vi "))Channel.vi"(0 "channel in":T2, 1 "last element in":bool, 2 "This VI":refnum<vi>, 5 "valid":bool=TRUE, 7 "channelOp":T3, 9 "event priority (norm)":T1=enum."normal priority", 11 "msg in":cluster{"cmd":string, "data":variant}, 12 "abort in":bool, 13 "# event structures":u16=2) -> (3 "last element out":bool, 4 "channel out":T2, 6 "Event Registration Refnum":refnum<event-registration>[](array[refnum]), 8 "This VI out":refnum<vi>, 14 "aborted?":bool)   [LabVIEW 2019, in "Cmd-Data Event Messenger.lvlib"]
uses:
  Cmd-Data Event Messenger.lvlib
  EventMessengerData.lvclass/EventMessengerData.ctl
  Instantiate.vi
  EventMessengerData.lvclass
  <vilib>/event_ctls.llb/usereventprio.ctl
  ))Channel.ctl
  ChannelOp.ctl
  Event Data.ctl
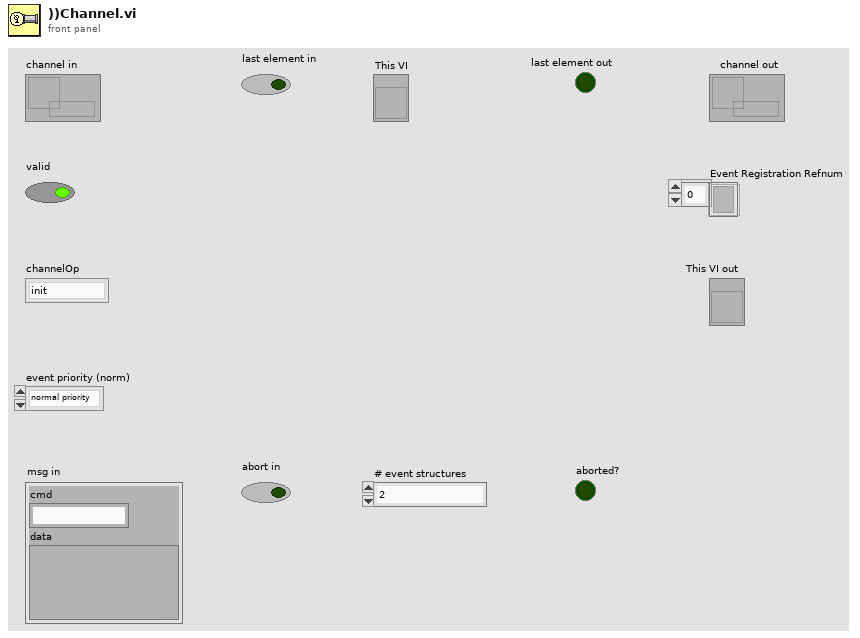
[diagram p1: front panel]
types:
  T1 = typedef "usereventprio.ctl" = enum32{"high priority", "normal priority"}
  T2 = typedef "Cmd-Data Event Messenger.lvlib/))Channel.ctl" = refnum<queue>
  T3 = typedef "Cmd-Data Event Messenger.lvlib/ChannelOp.ctl" = enum16{"init", "write", "register", "replicate", "probe"}
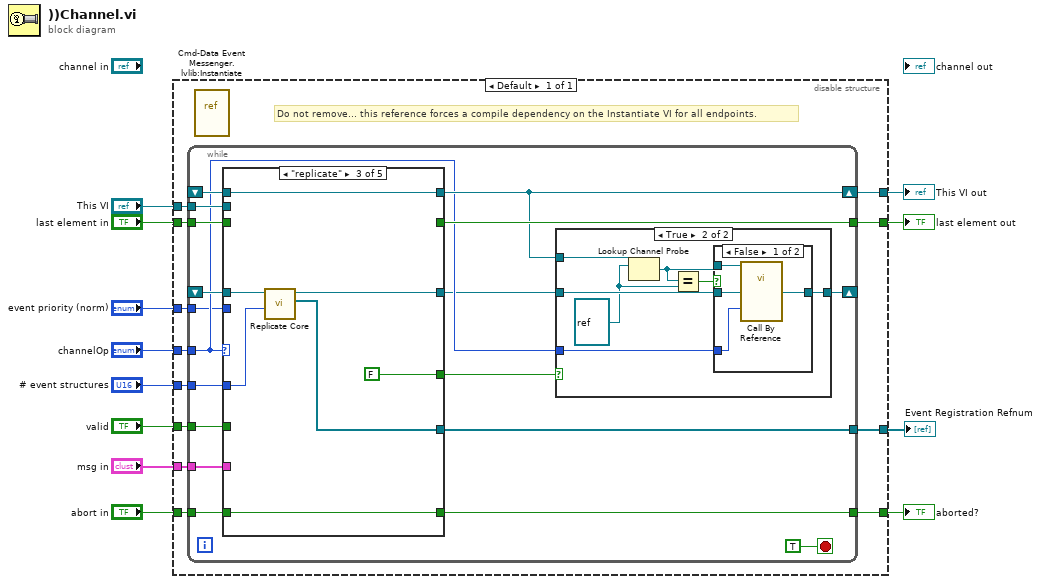
[diagram p0: block diagram]
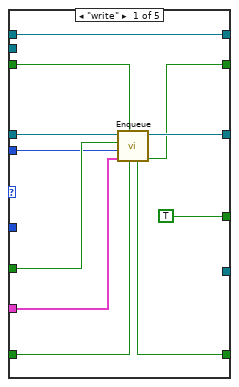
[diagram p4: hidden frame]
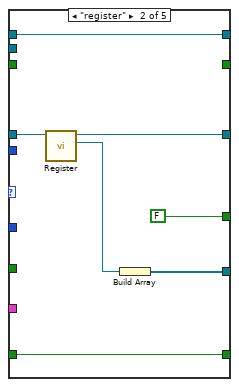
[diagram p5: hidden frame]
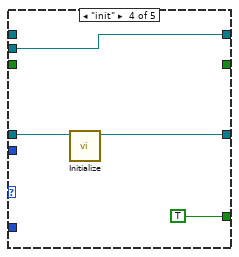
[diagram p6: hidden frame]
diagram:
  n1 = disable-structure shown="Default" {
    disable-tunnel: "msg in" -> [w24]
    disable-tunnel: "channelOp" -> [w23]
    disable-tunnel: "last element in" -> [w22]
    disable-tunnel: [w21] -> w9
    disable-tunnel: "valid" -> [w20]
    disable-tunnel: "abort in" -> [w19]
    disable-tunnel: [w18] -> w6
    disable-tunnel: "This VI" -> [w17]
    disable-tunnel: [w16] -> w4
    disable-tunnel: "event priority (norm)" -> [w15]
    disable-tunnel: "# event structures" -> [w14]
    disable-tunnel: [w13] -> w1
    frame Enabled {
      # "Do not remove... this reference forces a compile dependency on the Instantiate VI for all endpoints."
      n2 = while {
        shift-left: _ -> [w39]
        shift-right: [w32] -> _
        tunnel: w23 -> [w30]
        tunnel: w22 -> [w42]
        tunnel: [w41] -> w21
        tunnel: w20 -> [w38]
        tunnel: w19 -> [w37]
        tunnel: [w36] -> w18
        tunnel: w17 -> [w35]
        shift-right: [w33] -> w16
        shift-left: _ -> [w34]
        tunnel: w24 -> [w29]
        tunnel: [w28] -> w13
        tunnel: w15 -> [w26]
        tunnel: w14 -> [w25]
        stop <- TRUE stop-if-true
        n3 = case shown="\"replicate\"" w30 {
          tunnel: w29 -> [w64 _ _ _ _]
          tunnel: w42 -> [w58 _ _ _ _]
          tunnel: [w57 _ _ _ _] -> w41
          tunnel: [w65 w72 w76 w83 w86] -> w27
          tunnel: w39 -> [w66 w73 w77 w84 w86]
          tunnel: w38 -> [w63 _ _ _ _]
          tunnel: w37 -> [w62 w69 w78 _ _]
          tunnel: [w61 w69 w78 _ _] -> w36
          tunnel: w35 -> [_ _ _ w82 _]
          tunnel: [w60 w71 w80 w82 w85] -> w33
          tunnel: w34 -> [w60 w71 w80 _ w85]
          tunnel: [TRUE ("not an occurrence?") FALSE ("not an occurrence?") FALSE ("not an occurrence?") TRUE _] -> w31
          tunnel: [_ w67 w75 _ _] -> w28
          tunnel: w26 -> [w56 _ _ _ _]
          tunnel: w25 -> [_ _ w74 _ _]
          frame "write" {
            n4 = call "Enqueue.vi"("abort? (F)"=w62, "last element? (F)"=w58, "msg"=w64, "event priority"=w56, "is valid? (T)"=w63, "data in"=w66) -> ("last element?"=w57:bool, "data out"=w65:refnum<class "EventMessengerData.lvclass">, "aborted?"=w61:bool)  [unwired: 3 in]
          }
          frame "register" {
            n5 = call "Register.vi"("data in"=w73) -> ("Event Registration Refnum"=w68:refnum<event-registration>, "data out"=w72:refnum<class "EventMessengerData.lvclass">)  [unwired: 9 in]
            n6 = Build Array(w68) -> (w67:refnum<event-registration>[])
          }
          frame "replicate" {
            n7 = call "Replicate Core.vi"("# event structures"=w74, "data in"=w77) -> ("Event Registration Refnum"=w75:refnum<event-registration>[], "data out"=w76:refnum<class "EventMessengerData.lvclass">)  [unwired: 8 in]
          }
          frame "init" {
            n8 = call "Initialize.vi"("data in"=w84) -> ("data out"=w83:refnum<class "EventMessengerData.lvclass">)  [unwired: 9 in, 1 out]
          }
          frame "probe" {
            # "Probe case only exists to get the This VI Out."
          }
        }
        n9 = case shown="True" w31 {
          tunnel: w33 -> [_ w46]
          tunnel: w27 -> [w43 w49]
          tunnel: [w43 w48] -> w32
          tunnel: w30 -> [_ w47]
          frame False {
          }
          frame True {
            w44 = refnum<vi> refnum ("probe type specifier")
            n10 = Lookup Channel Probe(0:w46, 1:w44) -> (9:w45:refnum<vi>)  [unwired: 1 in, 1 out]
            n11 = Equal?(x=w45, y=w44) -> (x = y?=w50:bool)
            n12 = case shown="False" w50 {
              tunnel: w45 -> [w53 _]
              tunnel: w49 -> [w51 w55]
              tunnel: [w54 w55] -> w48
              tunnel: w47 -> [w52 _]
              frame False {
                n13 = call-by-ref "?"(reference=w53, "channelOp"=w52, "data in"=w51) -> ("data out"=w54:refnum<class "EventMessengerData.lvclass">)  [unwired: 2 in, 2 out]
              }
              frame True {
              }
            }
          }
        }
      }
      n14 = vi-ref "Cmd-Data Event Messenger.lvlib:Instantiate.vi"() -> ()  [unwired: 1 out]
    }
  }
  "last element out" <- w9
  "aborted?" <- w6
  "This VI out" <- w4
  "Event Registration Refnum" <- w1
